vi "Schedule Periodic Message.vi"(8 "error in":errorcluster, 11 "Chronometer in":refnum<class "Chronometer.lvclass">) -> (0 "error out":errorcluster, 3 "Chronometer out":refnum<class "Chronometer.lvclass">)   [LabVIEW 2023, in "Chronometer.lvlib" / "Chronometer.lvclass"]
uses:
  Chronometer.lvclass
  C:/Users/Public/Documents/Development/builds/Engine/Engine.lvlibp/Project/Engine.lvclass
  Chronometer Messages/Cumulate Time Msg/Cumulate Time Msg.lvclass
  C:/Users/Public/Documents/Development/builds/Engine/Actor Framework.lvlibp/1abvi3w/vi.lib/ActorFramework/Message/Message.lvclass
  Chronometer Messages/Update Record Msg/Update Record Msg.lvclass
  Chronometer.lvclass/Chronometer.ctl
  builds/Engine/Engine.lvlibp/Accessors/Read Self Q.vi
  builds/Engine/Actor Framework.lvlibp/1abvi3w/vi.lib/ActorFramework/Message Enqueuer/Message Enqueuer.lvclass
  builds/Engine/Actor Framework.lvlibp
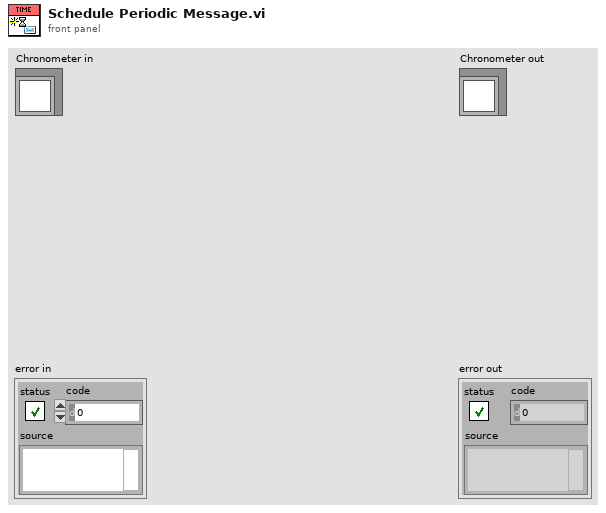
[diagram p1: front panel]
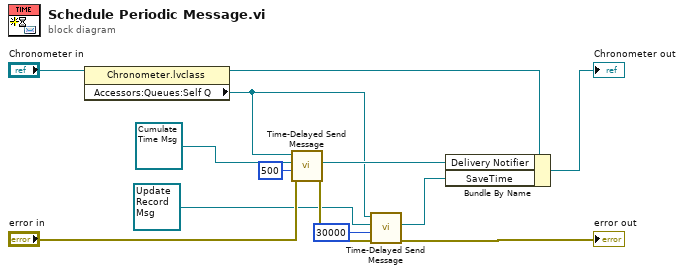
[diagram p0: block diagram]
diagram:
  n1 = property class="Chronometer.lvclass"(reference="Chronometer in") -> (reference out=w7:refnum<class "Chronometer.lvclass">, "Accessors:Queues:Self Q"=w1:refnum<class "Message Enqueuer.lvclass">)  [unwired: 1 in, 1 out]
  n2 = call "Time-Delayed Send Message.vi"("error in (no error)"="error in", "Milliseconds To Wait"=500, "Message"=refnum<class "Cumulate Time Msg.lvclass"> refnum ("Chronometer.lvlib:Cumulate Time Msg.lvclass"), "Message Enqueuer"=w1) -> ("error out"=w6:errorcluster, "Delivery Notifier"=w10:refnum<notifier>)  [unwired: 6 in]
  n3 = call "Time-Delayed Send Message.vi"("error in (no error)"=w6, "Milliseconds To Wait"=30000, "Message"=refnum<class "Update Record Msg.lvclass"> refnum ("Chronometer.lvlib:Update Record Msg.lvclass"), "Message Enqueuer"=w1) -> ("error out"=→"error out":errorcluster, "Delivery Notifier"=w2:refnum<notifier>)  [unwired: 6 in]
  n4 = Bundle By Name(cluster=w7, "Delivery Notifier"=w10, "SaveTime"=w2) -> (→"Chronometer out":refnum<class "Chronometer.lvclass">)
